vi "UDP Shot Detector.vi"() -> ()   [LabVIEW 2017]
uses:
  Global 1.vi
panel:
  out "number":i32
  out "data out":string
  in  "Stop":bool
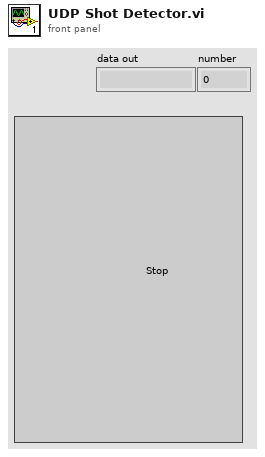
[diagram p1: front panel]
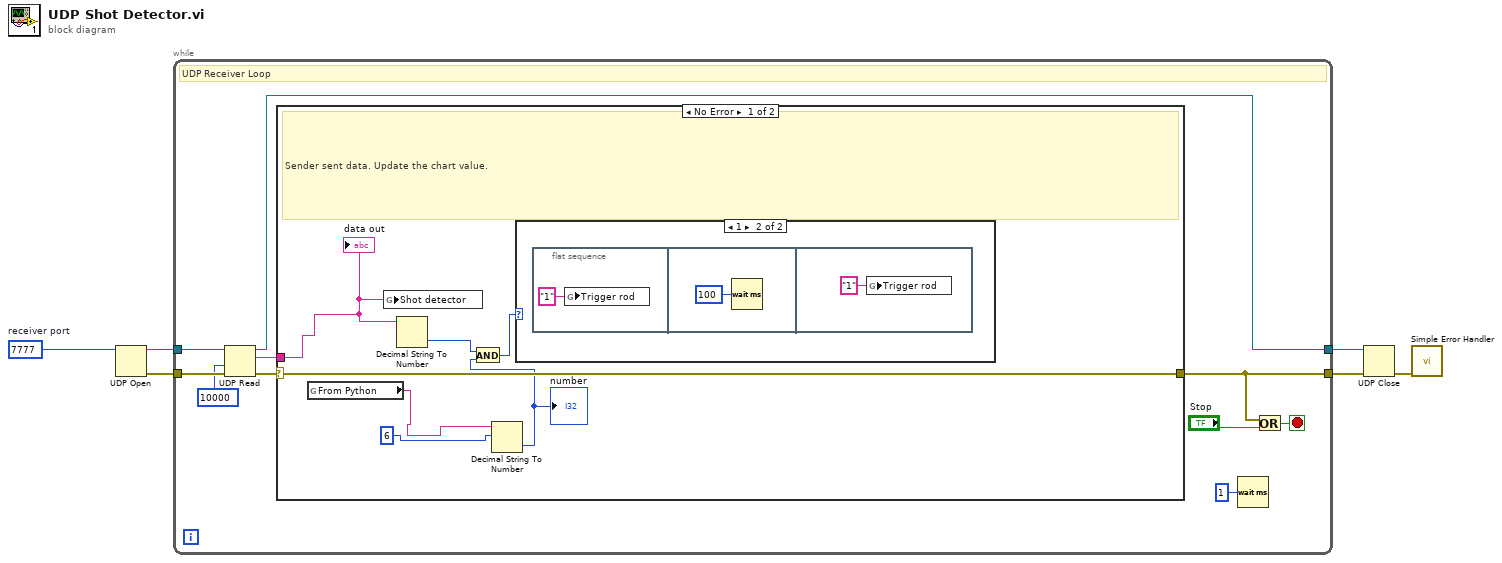
[diagram p0: block diagram]
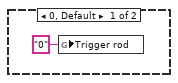
[diagram p2: hidden frame]
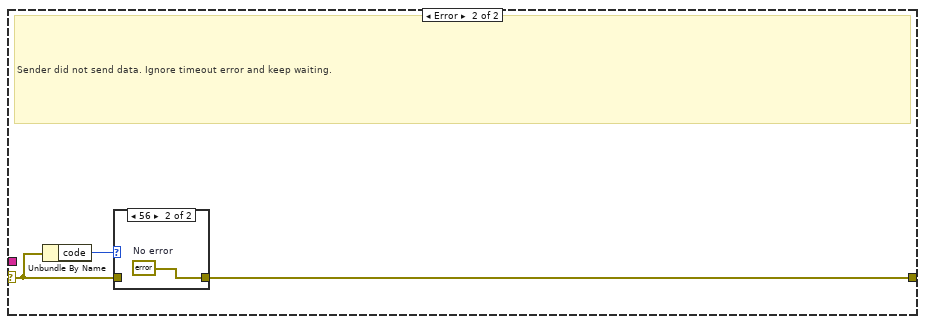
[diagram p3: hidden frame]
diagram:
  w1 = u16 7777  # receiver port
  n1 = UDP Open(11:w1) -> (port=w2:refnum<k16>, 0:w3:errorcluster)  [unwired: 4 in, 1 out]
  n2 = while {
    tunnel: w2 -> [w16]
    tunnel: [w8] -> w6
    tunnel: w3 -> [w13]
    tunnel: [w9] -> w4
    stop <- w14 stop-if-true
    # "UDP Receiver Loop"
    n3 = UDP Read(connection ID=w16, timeout ms (25000)=10000, 8:w13) -> (data out=w11:string, error out=w10:errorcluster, 3:w8:refnum<k16>)  [unwired: 3 out]
    n4 = case shown="No Error" w10 {
      selector: w10 -> [w23 w29]
      tunnel: w11 -> [w19 _]
      tunnel: [w23 w28] -> w9
      frame No Error {
        # "Sender sent data. Update the chart value."
        n5 = global read "Global 1.vi" "From Python"() -> (w17:string)
        n6 = global write "Global 1.vi" "Shot detector"(w19) -> ()
        n7 = Decimal String To Number(string=w19) -> (number=w21:i32)  [unwired: 2 in, 1 out]
        n8 = Decimal String To Number(string=w17, offset=6 ("offset (0)")) -> (number=w22:i32)  [unwired: 1 in, 1 out]
        "number" <- w22
        n9 = And(x=w21, y=w22) -> (x .and. y?=w20:i32)
        n10 = case shown="1" w20 {
          frame 0, Default {
            n11 = global write "Global 1.vi" "Trigger rod"("0" ("Trigger rod")) -> ()
          }
          frame 1 {
            n12 = flat-sequence {
              frame #0 {
                n13 = global write "Global 1.vi" "Trigger rod"("1" ("Trigger rod")) -> ()
              }
              frame #1 {
                n14 = Wait (ms)(milliseconds to wait=u32 100) -> ()  [unwired: 1 out]
              }
              frame #2 {
                n15 = global write "Global 1.vi" "Trigger rod"("1" ("Trigger rod")) -> ()
              }
            }
          }
        }
        "data out" <- w19
      }
      frame Error {
        # "Sender did not send data. Ignore timeout error and keep waiting."
        n16 = Unbundle By Name(w29) -> ("code"=w30:i32)
        n17 = case shown="56" w30 {
          tunnel: w29 -> [w31 _]
          tunnel: [w31 w32] -> w28
          frame Default {
          }
          frame 56 {
            w32 = errorcluster {"status"=FALSE, "code"=0, "source"=""}  # No error
          }
        }
      }
    }
    n18 = Wait (ms)(milliseconds to wait=u32 1) -> ()  [unwired: 1 out]
    n19 = Or(x=w9, y="Stop") -> (x .or. y?=w14:bool)
  }
  n20 = UDP Close(connection ID=w6, 8:w4) -> (error out=w5:errorcluster)  [unwired: 1 out]
  n21 = call <vilib>:"Simple Error Handler.vi"("error in (no error)"=w5) -> ()  [unwired: 1 in, 8 out]
